vi "Global 1.vi"() -> ()   [LabVIEW 2018]
panel:
  in  "Hatch Lift Power":dbl
  in  "Manual Elevator Mode?":bool
  in  "Turbo Drive Power":dbl
  in  "Slow Drive Power":dbl
  in  "Elevator Power":dbl
  out "Level Indicator":dbl
  in  "Top Level":bool
  in  "Level 2":bool
  in  "Level 1":bool
  in  "Floor Level":bool
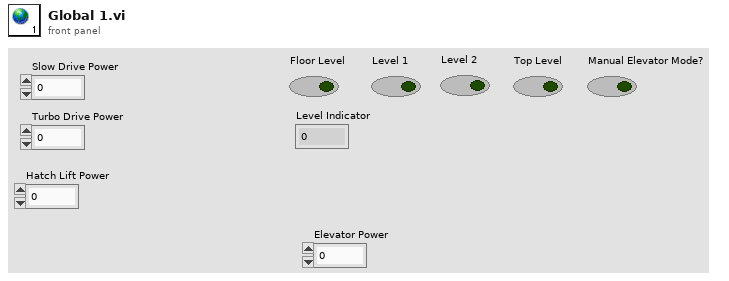
[diagram p1: front panel]
diagram:
